vi "max_tq_choose.vi"(9 "max torque in":dbl, 10 "Torque":dbl, 11 "max tq offset":bool) -> (3 "max torque out":dbl)   [LabVIEW 2014]
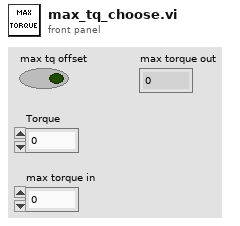
[diagram p1: front panel]
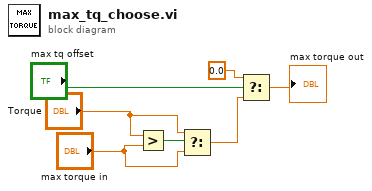
[diagram p0: block diagram]
diagram:
  n1 = Greater?(x="Torque", y="max torque in") -> (0:w7:bool)
  n2 = Select(t="Torque", s=w7, f="max torque in") -> (s? t:f=w1:dbl)
  n3 = Select(t=0.0, s="max tq offset", f=w1) -> (s? t:f=→"max torque out":dbl)
